vi "Gateway_ResetSSH.vi"(8 "error in (no error)":errorcluster, 11 "GatewayClass in":refnum<class "GatewayClass.lvclass">) -> (0 "error out":errorcluster, 3 "GatewayClass out":refnum<class "GatewayClass.lvclass">)   [LabVIEW 2018, in "GatewayClass.lvclass"]
uses:
  GatewayClass.lvclass
  DataPacker/Utilities/SSH_TUNNEL.lvclass
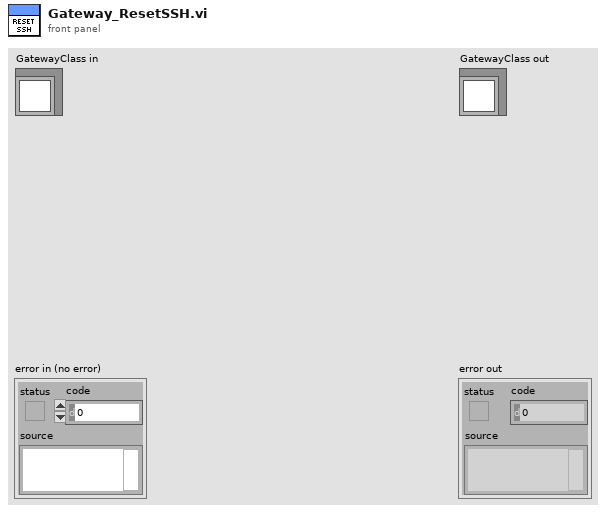
[diagram p1: front panel]
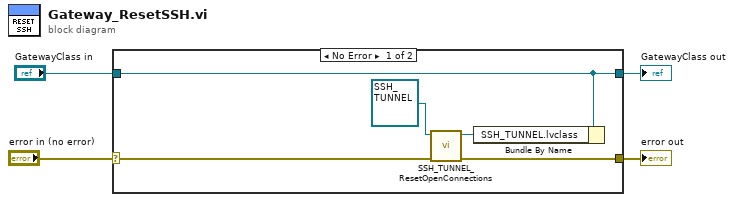
[diagram p0: block diagram]
diagram:
  n1 = case shown="No Error" "error in (no error)" {
    selector: "error in (no error)" -> [w6 w11]
    tunnel: [w5 w11] -> w3
    tunnel: [w9 w10] -> w1
    tunnel: "GatewayClass in" -> [w9 w10]
    frame No Error {
      n2 = call "SSH_TUNNEL_ResetOpenConnections.vi"("error in (no error)"=w6, "SSH_TUNNEL in"=refnum<class "SSH_TUNNEL.lvclass"> refnum ("SSH_TUNNEL.lvclass")) -> ("error out"=w5:errorcluster, "SSH_TUNNEL out"=w7:refnum<class "SSH_TUNNEL.lvclass">)  [unwired: 8 in]
      n3 = Bundle By Name(cluster=w9, "SSH_TUNNEL.lvclass"=w7) -> ()  [unwired: 1 out]
    }
    frame Error {
    }
  }
  "error out" <- w3
  "GatewayClass out" <- w1
